vi "Get Output Limits.vi"(8 "error in (no error)":errorcluster, 10 "Set Limits (T: Voltage)":bool=TRUE, 11 "VISA resource name":refnum<visa-resource-name>) -> (0 "error out":errorcluster, 1 "Positive Limit Value":dbl format="%^.3e", 2 "Negative Limit Value":dbl format="%^.3e", 3 "VISA resource name out":refnum<visa-resource-name>)   [LabVIEW 2011, in "Fluke 5XXX Series Multicalibrators.lvlib"]
doc: "This VI returns the maximum permissible output magnitude, negative and positive, for voltage and current, which is saved in the Calibrator non-volatile memory."
uses:
  Fluke 5XXX Series Multicalibrators.lvlib
panel:
  # "Voltage"
  # "Current"
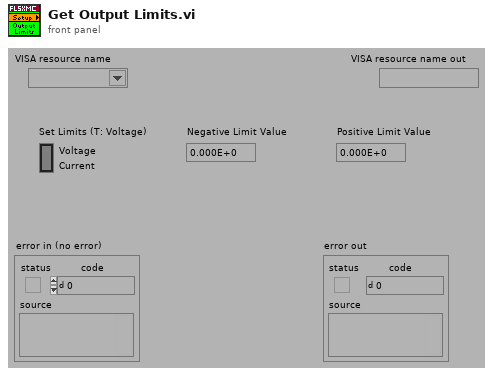
[diagram p1: front panel]
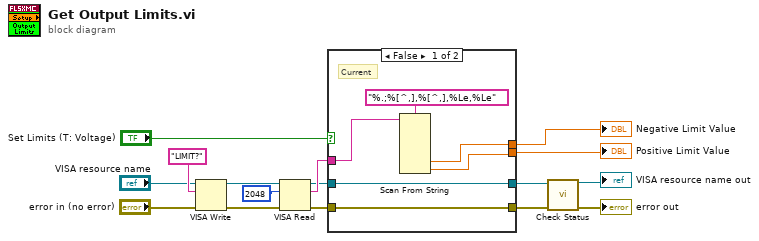
[diagram p0: block diagram]
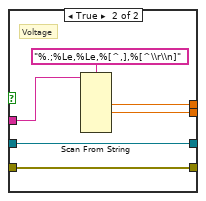
[diagram p2: hidden frame]
diagram:
  n1 = VISA Write(VISA resource name="VISA resource name", write buffer="LIMIT?", error in (no error)="error in (no error)") -> (VISA resource name out=w15:refnum<visa-resource-name>, error out=w14:errorcluster)  [unwired: 1 out]
  n2 = VISA Read(VISA resource name=w15, byte count=u32 2048 ("byte count (0)"), error in (no error)=w14) -> (VISA resource name out=w8:refnum<visa-resource-name>, read buffer=w12:string, error out=w11:errorcluster)  [unwired: 1 out]
  n3 = case shown="False" "Set Limits (T: Voltage)" {
    tunnel: w12 -> [w21 w27]
    tunnel: w11 -> [w20 w25]
    tunnel: [w20 w25] -> w10
    tunnel: [w19 w26] -> w9
    tunnel: w8 -> [w19 w26]
    tunnel: [w17 w24] -> w2
    tunnel: [w18 w23] -> w1
    frame False {
      # "Current"
      n4 = Scan From String(format string="%.;%[^,],%[^,],%Le,%Le", input string=w21) -> (output 3=w17:dbl, output 4=w18:dbl)  [unwired: 8 in, 3 out]
    }
    frame True {
      # "Voltage"
      n5 = Scan From String(format string="%.;%Le,%Le,%[^,],%[^\\r\\n]", input string=w27) -> (output 1=w24:dbl, output 2=w23:dbl)  [unwired: 8 in, 3 out]
    }
  }
  "Negative Limit Value" <- w2
  "Positive Limit Value" <- w1
  n6 = call "Check Status.vi"("VISA resource name"=w9, "error in (no error)"=w10) -> ("VISA resource name out"=→"VISA resource name out":refnum<visa-resource-name>, "error out"=→"error out":errorcluster)  [unwired: 12 in]
